vi "Play Sound.vi"(8 "error in (no error)":errorcluster, 9 "Enable Sound":bool, 10 "Volume":dbl(knob) scale=0.0..2000.0, 11 "Electrophysiology in":refnum<class "Electrophysiology.lvclass">) -> (0 "error out":errorcluster, 3 "Electrophysiology out":refnum<class "Electrophysiology.lvclass">)   [LabVIEW 2014, in "Electrophysiology.lvclass"]
uses:
  Electrophysiology.lvclass
  Electrophysiology.lvclass/Electrophysiology.ctl
  <vilib>/sound2/lvsound2.llb/Sound Output Write (DBL).vi
panel:
  in  "Recharge pause":u32=100
  in  "Max Backlog":i32=5
  out "Backlog error":dbl
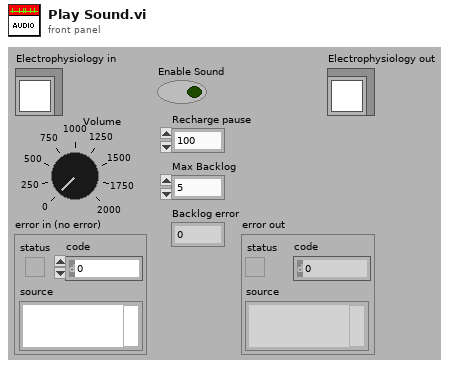
[diagram p1: front panel]
types:
  T1 = typedef "Sound Output Task ID.ctl" = u32
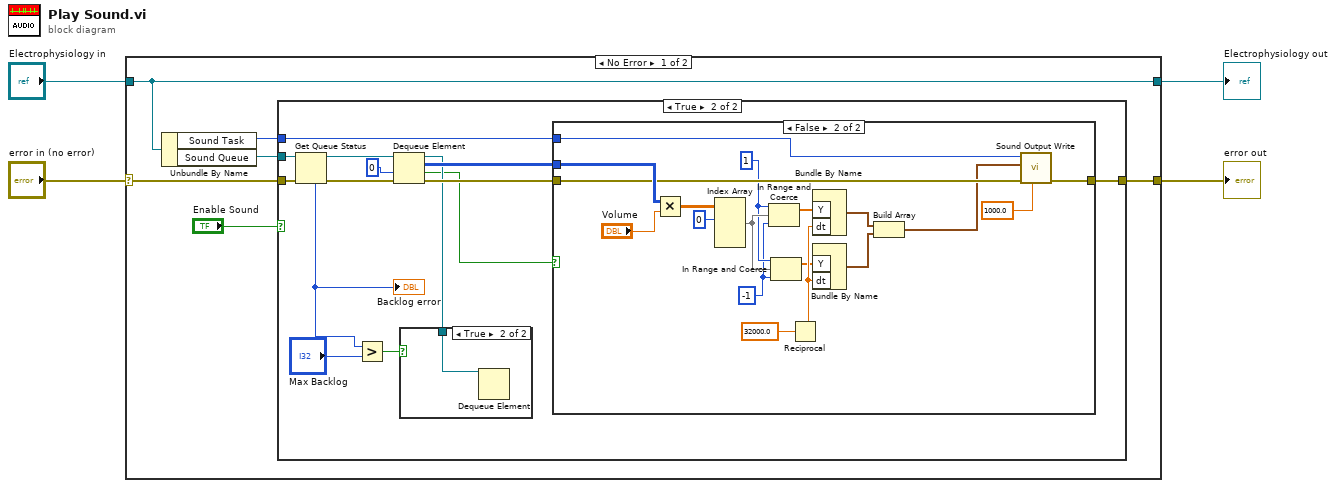
[diagram p0: block diagram]
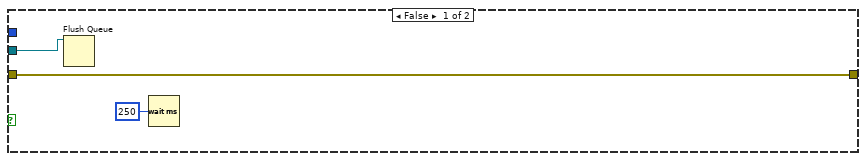
[diagram p2: hidden frame]
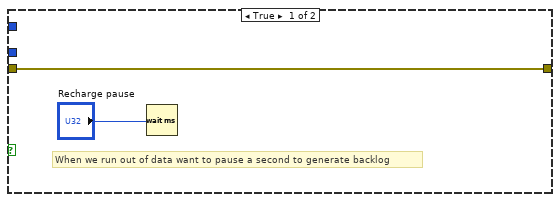
[diagram p3: hidden frame]
diagram:
  n1 = case shown="No Error" "error in (no error)" {
    selector: "error in (no error)" -> [w8 w50]
    tunnel: [w7 w50] -> w3
    tunnel: [w10 w49] -> w1
    tunnel: "Electrophysiology in" -> [w10 w49]
    frame No Error {
      n2 = Unbundle By Name(w10) -> ("Sound Task"=w9:T1, "Sound Queue"=w6:refnum<queue>)
      n3 = case shown="True" "Enable Sound" {
        tunnel: w9 -> [_ w27]
        tunnel: w8 -> [w13 w20]
        tunnel: [w13 w26] -> w7
        tunnel: w6 -> [w11 w22]
        frame False {
          n4 = Flush Queue(queue=w11) -> ()  [unwired: 1 in, 3 out]
          n5 = Wait (ms)(milliseconds to wait=u32 250) -> ()  [unwired: 1 out]
        }
        frame True {
          n6 = Get Queue Status(queue=w22, error in (no error)=w20) -> (queue out=w21:refnum<queue>, error out=w19:errorcluster, # elements in queue=w15:i32)  [unwired: 1 in, 5 out]
          "Backlog error" <- w15
          n7 = Greater?(x=w15, y="Max Backlog") -> (0:w17:bool)
          n8 = Dequeue Element(queue=w21, timeout in ms (-1)=u32 0 ("milliseconds to wait"), error in (no error)=w19) -> (queue out=w16:refnum<queue>, element=w25:i32[][], timed out?=w14:bool, error out=w24:errorcluster)
          n9 = case shown="True" w17 {
            tunnel: w16 -> [_ w48]
            frame False {
            }
            frame True {
              n10 = Dequeue Element(queue=w48) -> ()  [unwired: 2 in, 4 out]
            }
          }
          n11 = case shown="False" w14 {
            tunnel: w27 -> [_ w47]
            tunnel: [w28 w46] -> w26
            tunnel: w25 -> [_ w45]
            tunnel: w24 -> [w28 w44]
            frame True {
              # "When we run out of data want to pause a second to generate backlog"
              n12 = Wait (ms)(milliseconds to wait="Recharge pause") -> ()  [unwired: 1 out]
            }
            frame False {
              w30 = -1
              w31 = 1
              n13 = Multiply(x=w45, y="Volume") -> (x*y=w41:dbl[][])
              n14 = Index Array(array=w41, index (row) #1=0 ("index (row)")) -> (element #1=w34:dbl[])  [unwired: 3 in, 1 out]
              n15 = In Range and Coerce(upper limit=w31, x=w34, lower limit=w30) -> (coerced(x)=w32:dbl[])  [unwired: 1 out]
              n16 = In Range and Coerce(upper limit=w31, x=w34, lower limit=w30) -> (coerced(x)=w33:dbl[])  [unwired: 1 out]
              n17 = Reciprocal(x=32000.0) -> (1/x=w42:dbl)
              n18 = Bundle By Name("Y"=w32, "dt"=w42) -> (w38:waveform(dbl))  [unwired: 1 in]
              n19 = Bundle By Name("Y"=w33, "dt"=w42) -> (w39:waveform(dbl))  [unwired: 1 in]
              n20 = Build Array(w38, w39) -> (w36:waveform(dbl)[])
              n21 = call-poly <vilib>:"Sound Output Write.vi"("timeout (sec)"=1000.0, "error in (no error)"=w44, "data"=w36, "task ID"=w47) -> ("error out"=w46:errorcluster)  [unwired: 6 in, 1 out]
            }
          }
        }
      }
    }
    frame Error {
    }
  }
  "error out" <- w3
  "Electrophysiology out" <- w1
